vi "Add Multiple.vi"(7 "Q Ref In":refnum<queue>, 8 "error in":errorcluster, 11 "Q Packets":T1(array[cluster])) -> (0 "error out":errorcluster, 5 "Q Ref Out":refnum<queue>)   [LabVIEW 2025, in "Q Wrappers.lvlib"]
uses:
  Q Wrappers.lvlib
  Q Packet.ctl
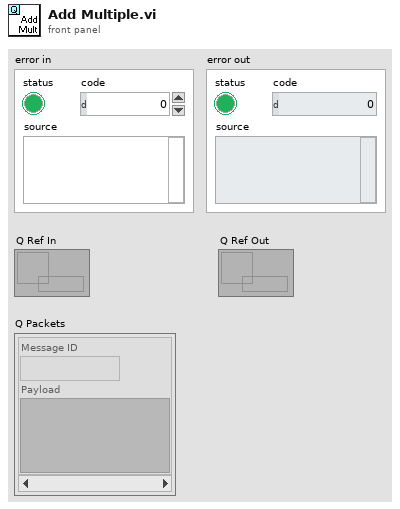
[diagram p1: front panel]
types:
  T1 = cluster{"Message ID":string, "Payload":variant}[]
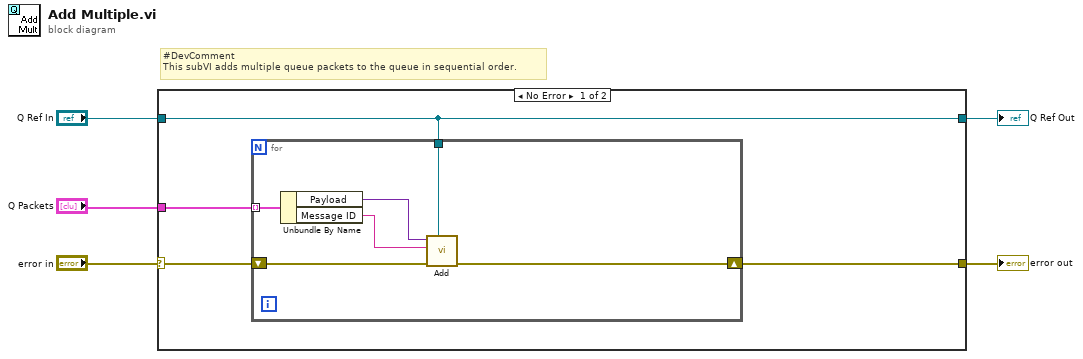
[diagram p0: block diagram]
diagram:
  # "#DevComment\nThis subVI adds multiple queue packets to the queue in sequential order."
  n1 = case shown="No Error" "error in" {
    selector: "error in" -> [w8 w16]
    tunnel: "Q Packets" -> [w9 _]
    tunnel: "Q Ref In" -> [w7 w17]
    tunnel: [w7 w17] -> w2
    tunnel: [w6 w16] -> w1
    frame No Error {
      n2 = for {
        tunnel: w9 -> [w14] mode=indexing
        tunnel: w7 -> [w11]
        shift-right: [w10] -> w6
        shift-left: w8 -> [w15]
        n3 = Unbundle By Name(w14) -> ("Payload"=w12:variant, "Message ID"=w13:string)
        n4 = call "Add.vi"("Q Ref In"=w11, "error in"=w15, "Message ID"=w13, "Payload"=w12) -> ("error out"=w10:errorcluster)  [unwired: 4 in, 3 out]
      }
    }
    frame Error {
    }
  }
  "error out" <- w1
  "Q Ref Out" <- w2
